vi "ArcadeScalePieceWise.vi"(11 "Direction":dbl) -> (3 "Scale":dbl)   [LabVIEW 2013]
panel:
  in  "Cutoff":dbl=0.3 format="%#_13g"
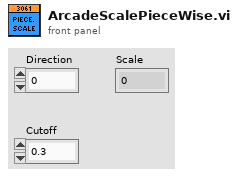
[diagram p1: front panel]
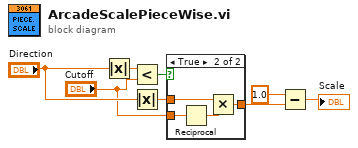
[diagram p0: block diagram]
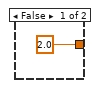
[diagram p2: hidden frame]
diagram:
  n1 = Absolute Value(x="Direction") -> (abs(x)=w8:dbl)
  n2 = Less?(x=w8, y="Cutoff") -> (x < y?=w7:bool)
  n3 = Absolute Value(x="Direction") -> (abs(x)=w4:dbl)
  n4 = case shown="True" w7 {
    tunnel: w4 -> [_ w12]
    tunnel: [2.0 w13] -> w5
    tunnel: "Cutoff" -> [_ w10]
    frame False {
    }
    frame True {
      n5 = Reciprocal(x=w10) -> (1/x=w11:dbl)
      n6 = Multiply(x=w12, y=w11) -> (x*y=w13:dbl)
    }
  }
  n7 = Subtract(x=1.0, y=w5) -> (x-y=→"Scale":dbl)
